vi "Edit_User.vi"(2 "用户ID":string) -> ()   [LabVIEW 2020]
uses:
  Global1.vi
  <vilib>/addons/database/Connection.llb/DB Tools Open Connec (String).vi
  <vilib>/addons/database/Connection.llb/Conn Execute.vi
  <vilib>/addons/database/Recordset.llb/Rec Fetch Recordset Data (R).vi
  <vilib>/addons/database/NI_Database_API.lvlib
panel:
  in  "取消":bool
  in  "保存":bool
  in  "用户权限":string(combo)="操作员"
  in  "员工编号":string
  in  "用户名":string
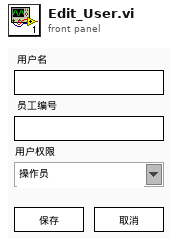
[diagram p1: front panel]
types:
  T1 = typedef "NI_Database_API.lvlib/Conn ObjectReference.ctl" = refnum<k1>
  T2 = typedef "NI_Database_API.lvlib/Rec ObjectReference.ctl" = refnum<k1>
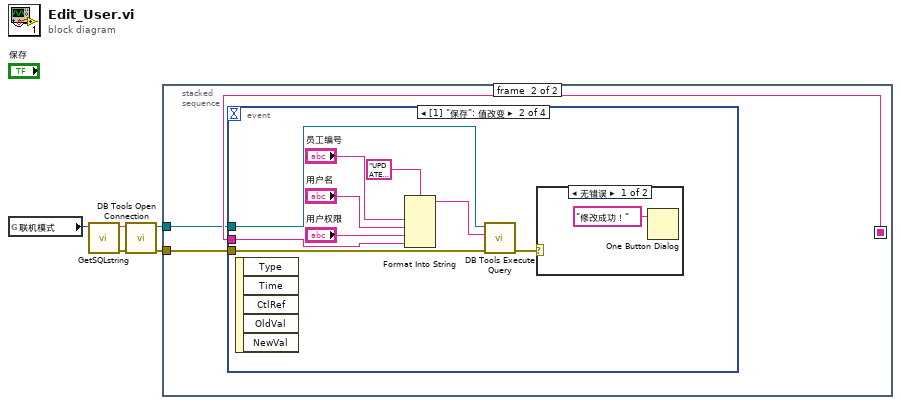
[diagram p0: block diagram]
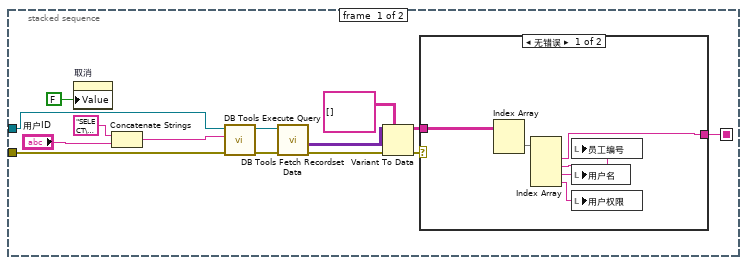
[diagram p2: hidden frame]
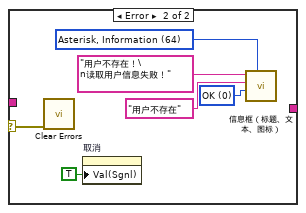
[diagram p3: hidden frame]
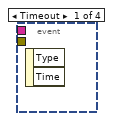
[diagram p4: hidden frame]
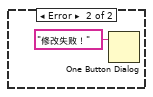
[diagram p5: hidden frame]
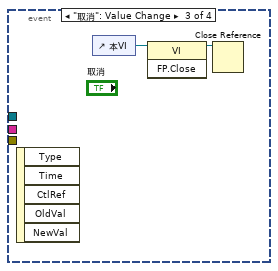
[diagram p6: hidden frame]
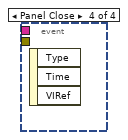
[diagram p7: hidden frame]
diagram:
  n1 = global read "Global1.vi" "联机模式"() -> (w3:enum16{"单机", "联网"})
  n2 = call "GetSQLstring.vi"("联机模式"=w3) -> ("错误输出"=w1:errorcluster, "连接字符串"=w2:string)  [unwired: 9 in]
  n3 = call-poly <vilib>:"DB Tools Open Connection.vi"("error in (no error)"=w1, "connection information"=w2) -> ("error out"=w4:errorcluster, "connection reference"=w5:T1)  [unwired: 6 in]
  n4 = stacked-sequence {
    seq-local: [w12 _] -> [_ w34]
    tunnel: w5 -> [w11 w33]
    tunnel: w4 -> [w10 w32]
    frame #0 {
      n5 = property on="取消" class="Bool (严格)"("Value"=FALSE ("取消")) -> ()  [unwired: 2 in, 2 out]
      n6 = Concatenate Strings("SELECT\ndbo.[User].USER_ID,\ndbo.[User].USER_EMPLOYEE_ID,\ndbo.[User].USER_NAME,\ndbo.[User].USER_PERMIT\n\nFROM\ndbo.[User]\n\nWHERE\ndbo.[user].USER_ID =\n" ("SQL query"), "用户ID") -> (w19:string)
      n7 = call-poly <vilib>:"DB Tools Execute Query.vi"("error in (no error)"=w10, "SQL query"=w19, "connection reference"=w11) -> ("error out"=w17:errorcluster, "recordset reference"=w18:T2)  [unwired: 5 in]
      n8 = call-poly <vilib>:"DB Tools Fetch Recordset Data.vi"("error in (no error)"=w17, "recordset reference"=w18) -> ("error out"=w16:errorcluster, "recordset data"=w15:variant[][])  [unwired: 3 in, 1 out]
      n9 = Variant To Data(error in=w16, type=string[][] [], Variant=w15) -> (data=w13:string[][], error out=w8:errorcluster)
      n10 = case shown="无错误" w8 {
        selector: w8 -> [_ w31]
        tunnel: w13 -> [w25 _]
        tunnel: [w20 _] -> w12
        frame No Error {
          n11 = Index Array(array=w25) -> (element=w24:string[])  [unwired: 2 in]
          n12 = Index Array(array=w24) -> (element #1=w20:string, element #2=w23:string, element #3=w22:string, element #4=w21:string)  [unwired: 4 in]
          n13 = local write "员工编号"(w23) -> ()
          n14 = local write "用户名"(w22) -> ()
          n15 = local write "用户权限"(w21) -> ()
        }
        frame Error {
          w27 = 64 items=["None"=0, "Hand, Error, Stop"=16, "Question"=32, "Exclamation, Warning"=48, "Asterisk, Information"=64] ("icon")
          w28 = 0 items=["OK", "OKCancel", "AbortRetryIgnore", "YesNoCancel", "YesNo", "RetryCancel"] ("buttons")
          n16 = call <vilib>:"Clear Errors.vi"("error in (no error)"=w31) -> ()  [unwired: 5 in, 2 out]
          n17 = property on="取消" class="Bool (严格)"("Val(Sgnl)"=TRUE) -> ()  [unwired: 2 in, 2 out]
          n18 = call "信息框（标题、文本、图标）.vi"("icon"=w27, "buttons"=w28, "caption"="用户不存在", "text"="用户不存在！\n读取用户信息失败！") -> ()  [unwired: 6 in, 2 out]
        }
      }
    }
    frame #1 {
      n19 = event shown="[1] \"保存\": 值改变" {
        selector: _ -> [_ _ _ _]
        dyn-events: _ -> [_ _ _ _]
        timeout: _ -> [_ _ _ _]
        tunnel: w34 -> [_ w43 _ _]
        tunnel: w33 -> [_ w39 _ _]
        tunnel: w32 -> [_ w37 _ _]
        event Timeout {
          n20 = event-data() -> ()  [unwired: 1 in, 2 out]
        }
        event "保存": Value Change {
          n21 = event-data() -> ()  [unwired: 1 in, 5 out]
          n22 = Format Into String(format string="UPDATE [dbo].[User] \nSET [USER_EMPLOYEE_ID]='%s', \n[USER_NAME]=N'%s',\n[USER_PERMIT]=N'%s' \nWHERE ([User_ID]=%s)", "员工编号", "用户名", "用户权限", w43) -> (resulting string=w38:string)  [unwired: 2 in, 1 out]
          n23 = call-poly <vilib>:"DB Tools Execute Query.vi"("error in (no error)"=w37, "SQL query"=w38, "connection reference"=w39) -> ("error out"=w36:errorcluster)  [unwired: 5 in, 1 out]
          n24 = case shown="无错误" w36 {
            frame No Error {
              n25 = One Button Dialog(message="修改成功！" ("消息")) -> ()  [unwired: 1 in, 1 out]
            }
            frame Error {
              n26 = One Button Dialog(message="修改失败！" ("消息")) -> ()  [unwired: 1 in, 1 out]
            }
          }
        }
        event "取消": Value Change {
          n27 = event-data() -> ()  [unwired: 1 in, 5 out]
          n28 = control-ref of="本VI"() -> (w47:refnum<vi>)
          n29 = invoke class="VI" method="FP.Close"(reference=w47) -> (reference out=w46:refnum<vi>)  [unwired: 2 in, 2 out]
          n30 = Close Reference(reference=w46) -> ()  [unwired: 1 in, 1 out]
        }
        event Panel Close {
          n31 = event-data() -> ()  [unwired: 1 in, 3 out]
        }
      }
    }
  }
